vi "Create-Obtain RT Queue.vi"(8 "error in (no error)":errorcluster) -> (0 "error out":errorcluster, 3 "Queue out":refnum<queue>)   [LabVIEW 2016]
uses:
  Controls/Message Structure.ctl
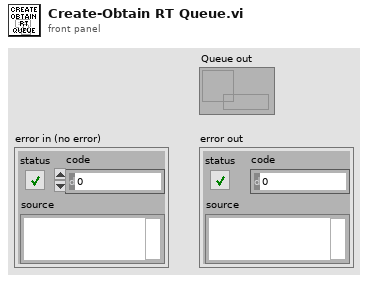
[diagram p1: front panel]
types:
  T1 = typedef "Message Structure.ctl" = cluster{"Data":variant, "Cmd":string}
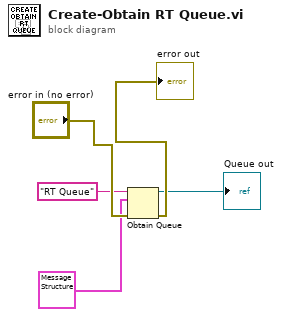
[diagram p0: block diagram]
diagram:
  n1 = Obtain Queue(name (unnamed)="RT Queue", element data type=T1 {"Data"=variant, "Cmd"=""}, error in (no error)="error in (no error)") -> (queue out=→"Queue out":refnum<queue>, error out=→"error out":errorcluster)  [unwired: 2 in, 1 out]
